vi "D Plotter Setup.vi"(5 "Address (5)":u32=5, 6 "Baud Rate(9600)":u32(ring)=3 items=["1200", "2400", "4800", "9600", "19200"], 7 "Port(Serial)":u16(ring)=1 items=["Parallel", "Serial", "GPIB"], 8 "error in (no error)":errorcluster, 9 "Type(Plotter:F)":bool, 10 "Handshake Mode(Xon-Xoff)":bool=TRUE, 11 "VISA resource name":refnum<visa-resource-name>) -> (0 "error out":errorcluster, 3 "VISA resource name out":refnum<visa-resource-name>)   [LabVIEW 2018, in "Agilent 87XX Series.lvlib"]
doc: "Sets up configuration information for the plotter. Only works on the HP8753D."
uses:
  Agilent 87XX Series.lvlib
panel:
  # "DTR-DSR"
  # "Xon-Xoff"
  # "HPGL-compatible printer"
  # "Plotter"
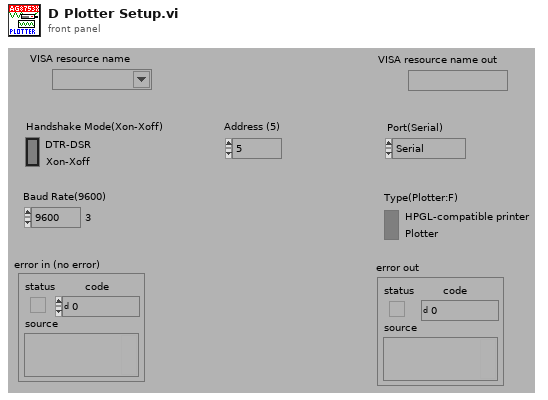
[diagram p1: front panel]
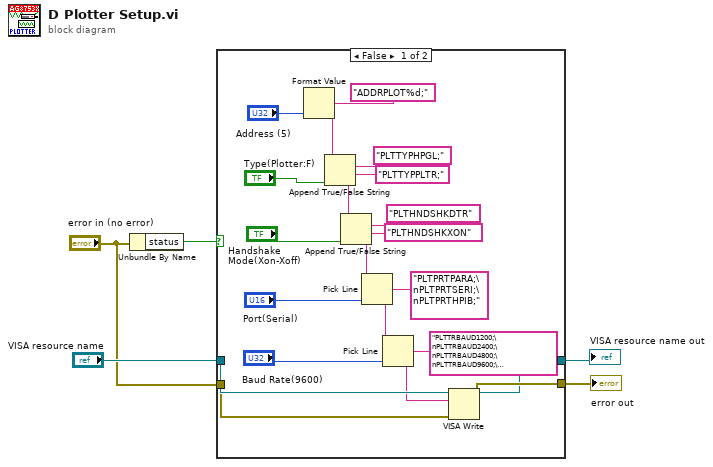
[diagram p0: block diagram]
diagram:
  n1 = Unbundle By Name("error in (no error)") -> ("status"=w5:bool)
  n2 = case shown="False" w5 {
    tunnel: [w26 w27] -> w4
    tunnel: "VISA resource name" -> [w25 w28]
    tunnel: "error in (no error)" -> [w24 w27]
    tunnel: [w23 w28] -> w1
    frame False {
      n3 = Format Value(format string="ADDRPLOT%d;", value (0)="Address (5)") -> (output string=w8:string)  [unwired: 1 in]
      n4 = Append True/False String(1:"Type(Plotter:F)", 2:"PLTTYPPLTR;", 3:"PLTTYPHPGL;", 4:w8) -> (0:w13:string)
      n5 = Append True/False String(1:"Handshake Mode(Xon-Xoff)", 2:"PLTHNDSHKXON", 3:"PLTHNDSHKDTR", 4:w13) -> (0:w12:string)
      n6 = Pick Line(string ("")=w12, multi-line string="PLTPRTPARA;\nPLTPRTSERI;\nPLTPRTHPIB;", line index="Port(Serial)") -> (output string=w20:string)
      n7 = Pick Line(string ("")=w20, multi-line string="PLTTRBAUD1200;\nPLTTRBAUD2400;\nPLTTRBAUD4800;\nPLTTRBAUD9600;\nPLTTRBAUD19200;", line index="Baud Rate(9600)") -> (output string=w9:string)
      n8 = VISA Write(VISA resource name=w25, write buffer=w9, error in (no error)=w24) -> (VISA resource name out=w23:refnum<visa-resource-name>, error out=w26:errorcluster)  [unwired: 1 out]
    }
    frame True {
    }
  }
  "VISA resource name out" <- w1
  "error out" <- w4
